vi "Receive Node Actor VI Ref.vi"(6 "Paras In":variant, 7 "System Actor In":refnum<class "System Actor.lvclass">, 8 "error in (no error)":errorcluster, 10 "VI Refnum":refnum<vi>, 11 "Simple Numeric Map Node Controller in":refnum<class "Simple Numeric Map Node Controller.lvclass">) -> (0 "error out":errorcluster, 3 "Simple Numeric Map Node Controller out":refnum<class "Simple Numeric Map Node Controller.lvclass">, 5 "System Actor Out":refnum<class "System Actor.lvclass">)   [LabVIEW 2024, in "Simple Numeric Map Node Controller.lvclass"]
uses:
  Simple Numeric Map Node Controller.lvclass
  Ancestor Class/Actor/System Actor/System Actor.lvclass
  Ancestor Class/Messenger/Mail Strategy/Mail Strategy.lvclass
  Ancestor Class/Actor/System Actor/System Actor.lvclass/System Actor.ctl
  Simple Numeric Map Node Controller.lvclass/Simple Numeric Map Node Controller.ctl
  Ancestor Class/Actor/System Actor/Public Data/Read ID.vi
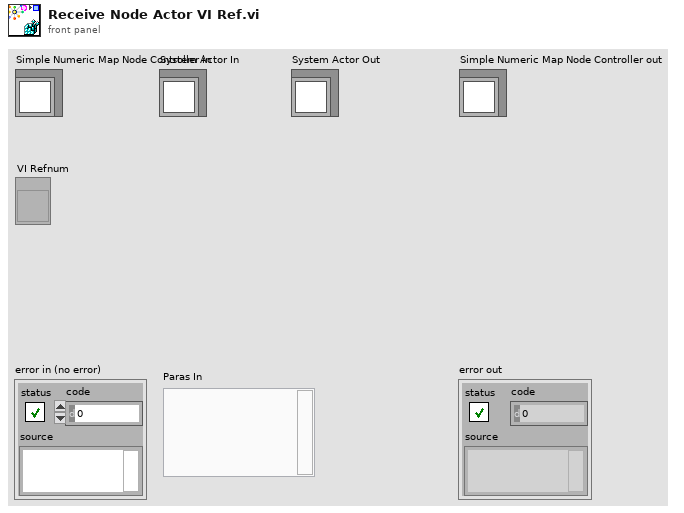
[diagram p1: front panel]
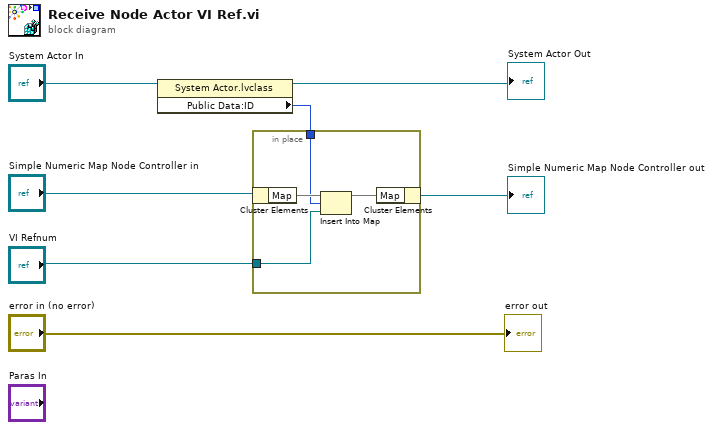
[diagram p0: block diagram]
diagram:
  n1 = property class="System Actor.lvclass"(reference="System Actor In") -> (reference out=→"System Actor Out":refnum<class "System Actor.lvclass">, "Public Data:ID"=w4:i64)  [unwired: 1 in, 1 out]
  n2 = in-place {
    in-place-border: w4 -> [w9]
    in-place-border: "VI Refnum" -> [w8]
    n3 = in-place-cluster #1("Simple Numeric Map Node Controller in") -> ("Map"=w11:map{i64, refnum<vi>})
    n4 = Insert Into Map(map in=w11, key=w9, value=w8) -> (map out=w10:map{i64, refnum<vi>})  [unwired: 2 out]
    n5 = in-place-cluster #1("Map"=w10) -> (→"Simple Numeric Map Node Controller out":refnum<class "Simple Numeric Map Node Controller.lvclass">)
  }
  "error out" <- "error in (no error)"
